vi "SA_GetPosition_S.vi"(5 "channelIndex":u32, 7 "systemIndex":u32, 8 "error in (no error)":errorcluster) -> (0 "error out":errorcluster, 3 "position":i32)   [LabVIEW 2013]
doc: "<B>Description:</B>\nReturns the current position of a positioner. This function is only executable by a positioner that has a sensor attached to it. The sensor must also be enabled or in power save mode (see SA_SetSensorEnabled_S). If this is not the case the channel will return an error. Additionally, the command is only executable if the addressed channel is configured to be of type linear (see SA_SetSensorType_S). A rotary channel will return an error.\n<B>Parameters:</B>\n<B>- systemIndex</B> (unsigned 32bit), input - Selects the system. The index is zero based.\n<B>- channelIndex</B> (unsigned 32bit), input - Selects the channel of the selected system. The index is zero based.\n<B>- position</B> (signed 32bit), output - If the call was successful this value holds the current position of the positioner in nano meters."
uses:
  MCSControl.dll
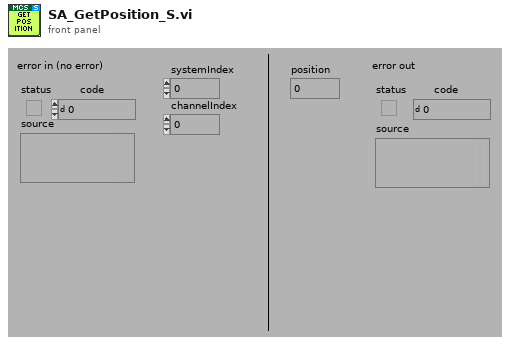
[diagram p1: front panel]
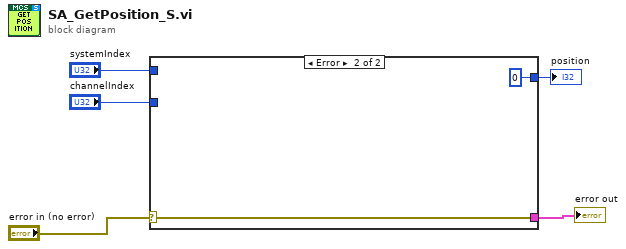
[diagram p0: block diagram]
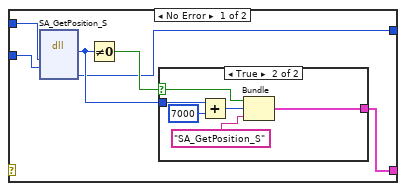
[diagram p2: hidden frame]
diagram:
  n1 = case shown="Error" "error in (no error)" {
    selector: "error in (no error)" -> [_ w19]
    tunnel: [w9 w19] -> w4
    tunnel: "systemIndex" -> [w8 _]
    tunnel: "channelIndex" -> [w7 _]
    tunnel: [w6 0 ("position")] -> w1
    frame No Error {
      n2 = dll-call lib="MCSControl.dll" fn="SA_GetPosition_S"("systemIndex"=w8, "channelIndex"=w7) -> (w10:u32, "position"=w6:i32)  [unwired: 6 in, 2 out]
      n3 = Not Equal To 0?(x=w10) -> (x != 0?=w11:bool)
      n4 = case shown="True" w11 {
        selector: w11 -> [_ w14]
        tunnel: w10 -> [_ w17]
        tunnel: [_ w12] -> w9
        frame False {
        }
        frame True {
          n5 = Add(x=w17, y=u32 7000) -> (x+y=w15:u32)
          n6 = Bundle(w14, w15, "source"="SA_GetPosition_S") -> (w12:cluster{bool, u32, "source":string})  [unwired: 1 in]
        }
      }
    }
    frame Error {
    }
  }
  "error out" <- w4
  "position" <- w1
